vi "read hdf timestamps.vi"(0 "file":string, 1 "start_index":i32, 2 "strideLength":i32, 5 "monitor_id":string, 7 "datasetName":string, 9 "data":cluster{}, 12 "nSamples":i32) -> (3 "function return":i32, 4 "file out":string, 6 "monitor_id out":string, 8 "datasetName out":string, 10 "data out":cluster{})   [LabVIEW 2019, in "apdm.lvlib"]
doc: "APDM_EXPORT int apdm_read_hdf_timestamps(char *file, char *monitor_id, char *datasetName, uint64_t *data, int start_index, int nSamples, int strideLength);"
uses:
  apdm.lvlib
  Lee Lab/CP FES Walking 2018/Code/Working/LabVIEW/apdm.dll
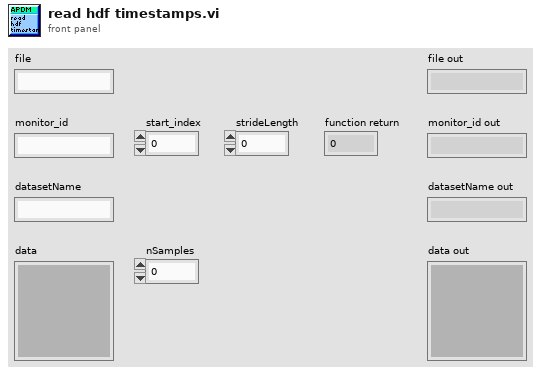
[diagram p1: front panel]
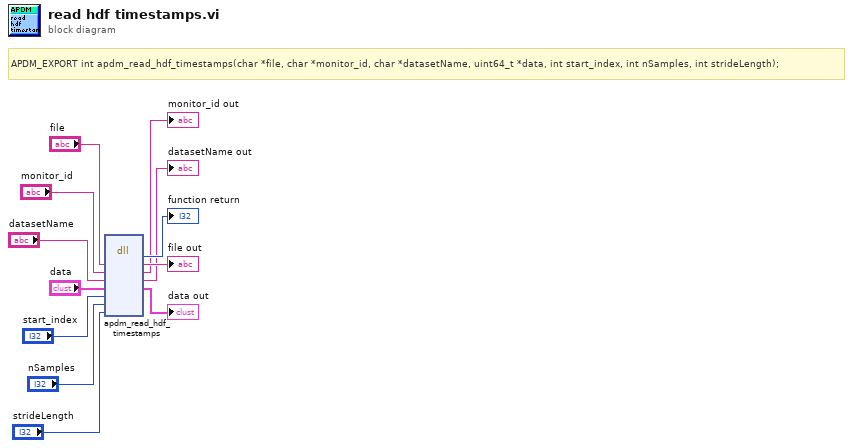
[diagram p0: block diagram]
diagram:
  # "APDM_EXPORT\tint apdm_read_hdf_timestamps(char *file, char *monitor_id, char *datasetName, uint64_t *data, int start_index, int nSamples, int strideLength);"
  n1 = dll-call lib="C:/Users/jfalesi/Dropbox/Lee Lab/CP FES Walking 2018/Code/Working/LabVIEW/apdm.*" fn="apdm_read_hdf_timestamps"("file"="file", "monitor_id"="monitor_id", "datasetName"="datasetName", "data"="data", "start_index"="start_index", "nSamples"="nSamples", "strideLength"="strideLength") -> (→"function return":i32, "file"=→"file out":string, "monitor_id"=→"monitor_id out":string, "datasetName"=→"datasetName out":string, "data"=→"data out":cluster{})  [unwired: 6 in, 2 out]
